vi "#33_MAV_MSG_GLOBAL_POSITION_INT_DECODE.vi"(11 "mavlink_payload":u8[](array[numeric])) -> (3 "GLOBAL_POSITION_INT":T1)   [LabVIEW 2023]
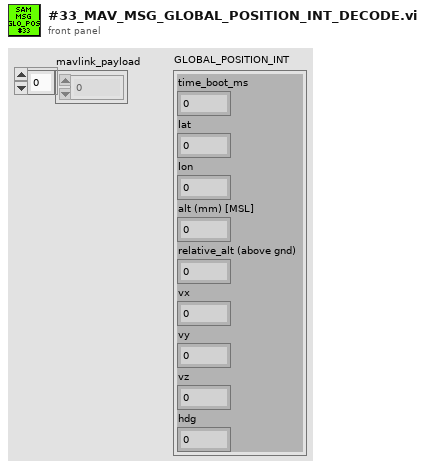
[diagram p1: front panel]
types:
  T1 = cluster{"time_boot_ms":u32, "lat":i32, "lon":i32, "alt (mm) [MSL]":i32, "relative_alt (above gnd)":i32, "vx":i16, "vy":i16, "vz":i16, "hdg":u16}
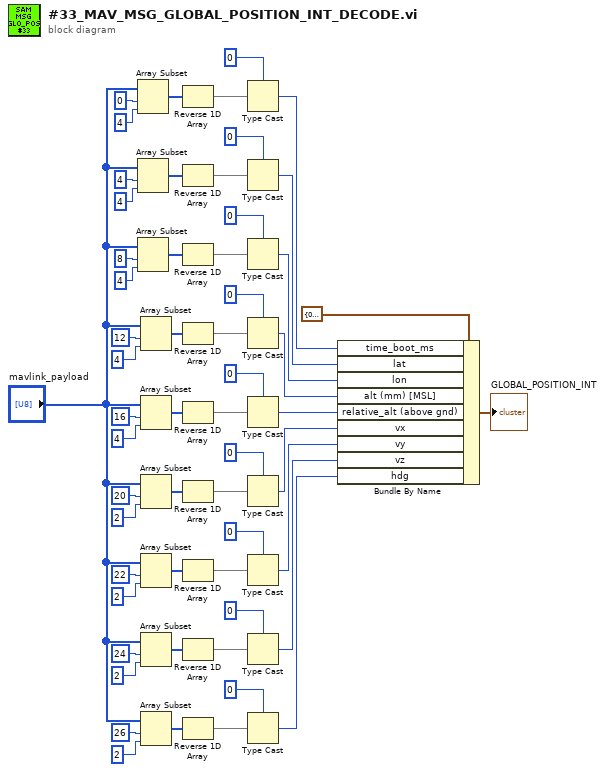
[diagram p0: block diagram]
diagram:
  n1 = Array Subset(array="mavlink_payload", index=0, length=4) -> (w57:u8[])
  n2 = Array Subset(array="mavlink_payload", index=4, length=4) -> (w49:u8[])
  n3 = Array Subset(array="mavlink_payload", index=8, length=4) -> (w44:u8[])
  n4 = Array Subset(array="mavlink_payload", index=12, length=4) -> (w37:u8[])
  n5 = Array Subset(array="mavlink_payload", index=16, length=4) -> (w31:u8[])
  n6 = Array Subset(array="mavlink_payload", index=20, length=2) -> (w25:u8[])
  n7 = Array Subset(array="mavlink_payload", index=22, length=2) -> (w19:u8[])
  n8 = Array Subset(array="mavlink_payload", index=24, length=2) -> (w13:u8[])
  n9 = Array Subset(array="mavlink_payload", index=26, length=2) -> (w7:u8[])
  n10 = Reverse 1D Array(array=w57) -> (reversed array=w56:u8[])
  n11 = Reverse 1D Array(array=w49) -> (reversed array=w48:u8[])
  n12 = Reverse 1D Array(array=w44) -> (reversed array=w43:u8[])
  n13 = Reverse 1D Array(array=w37) -> (reversed array=w36:u8[])
  n14 = Reverse 1D Array(array=w31) -> (reversed array=w30:u8[])
  n15 = Reverse 1D Array(array=w25) -> (reversed array=w24:u8[])
  n16 = Reverse 1D Array(array=w19) -> (reversed array=w18:u8[])
  n17 = Reverse 1D Array(array=w13) -> (reversed array=w12:u8[])
  n18 = Reverse 1D Array(array=w7) -> (reversed array=w6:u8[])
  n19 = Type Cast(type=u32 0, x=w56) -> (*(type *) &x=w52:u32)
  n20 = Type Cast(type=0, x=w48) -> (*(type *) &x=w39:i32)
  n21 = Type Cast(type=0, x=w43) -> (*(type *) &x=w38:i32)
  n22 = Type Cast(type=0, x=w36) -> (*(type *) &x=w32:i32)
  n23 = Type Cast(type=0, x=w30) -> (*(type *) &x=w26:i32)
  n24 = Type Cast(type=i16 0, x=w24) -> (*(type *) &x=w20:i16)
  n25 = Type Cast(type=i16 0, x=w18) -> (*(type *) &x=w14:i16)
  n26 = Type Cast(type=i16 0, x=w12) -> (*(type *) &x=w8:i16)
  n27 = Type Cast(type=u16 0, x=w6) -> (*(type *) &x=w1:u16)
  n28 = Bundle By Name(cluster=T1 {"time_boot_ms"=0, "lat"=0, "lon"=0, "alt (mm) [MSL]"=0, "relative_alt (above gnd)"=0, "vx"=0, "vy"=0, "vz"=0, "hdg"=0} ("GLOBAL_POSITION_INT"), "time_boot_ms"=w52, "lat"=w39, "lon"=w38, "alt (mm) [MSL]"=w32, "relative_alt (above gnd)"=w26, "vx"=w20, "vy"=w14, "vz"=w8, "hdg"=w1) -> (→"GLOBAL_POSITION_INT":T1)
